vi "Configure IQ vs Slot Measurement Filter.vi"(8 "error in (no error)":errorcluster, 9 "Filter Type (Gauss)":i32(ring) items=["Gauss", "Bandpass 1MHz", "Nyquist 1 MHz", "Bandpass 10MHz", "Nyquist 100kHz"], 10 "Instance (1)":i32=1 format="%.0g", 11 "VISA resource name":refnum<visa-resource-name>) -> (0 "error out":errorcluster, 3 "VISA resource name out":refnum<visa-resource-name>)   [LabVIEW 2015, in "Rohde&Schwarz CMXP GPRF.lvlib"]
doc: "Configures IQ vs Slot measurement filter type.\n\nAttribute:\nRSCMXPGPRF_ATTR_IQ_VS_SLOT_MEASUREMENT_FILTER_TYPE\n\nRemote-control command:\nCONFigure:GPRF:MEAS<i>:IQVSlot:FTYPe"
uses:
  <instrlib>/Rohde&Schwarz CMXP GPRF/Rohde&Schwarz CMXP GPRF.lvlib
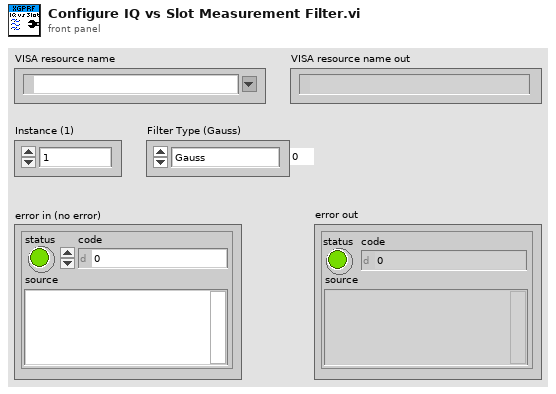
[diagram p1: front panel]
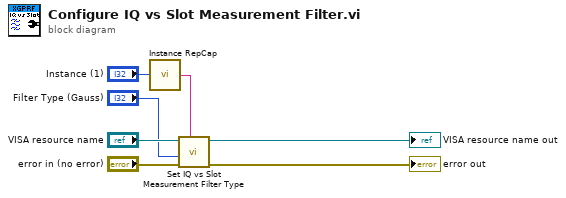
[diagram p0: block diagram]
diagram:
  n1 = call <instrlib>:"Instance RepCap.vi"("instance  in"="Instance (1)") -> ("instance out"=w7:string)
  n2 = call "Set IQ vs Slot Measurement Filter Type"("Repeated Capabilities"=w7, "error in (no error)"="error in (no error)", "IQ vs Slot Measurement Filter Type (0 - Gauss)"="Filter Type (Gauss)", "instrument handle"="VISA resource name") -> ("error out"=→"error out":errorcluster, "instrument handle out"=→"VISA resource name out":refnum<visa-resource-name>)  [unwired: 6 in]
